vi "New.vi"(7 "id (0)":i32, 8 "error in (no error)":errorcluster, 9 "priority (100)":i32=100, 10 "processor (-2)":i32=-2, 11 "Thread type":refnum<class "Thread.lvclass">) -> (0 "error out":errorcluster, 3 "Thread":refnum<class "Thread.lvclass">)   [LabVIEW 2017, in "DSF Core.lvlib" / "Thread.lvclass"]
uses:
  Thread.lvclass
  Thread.lvclass/Thread.ctl
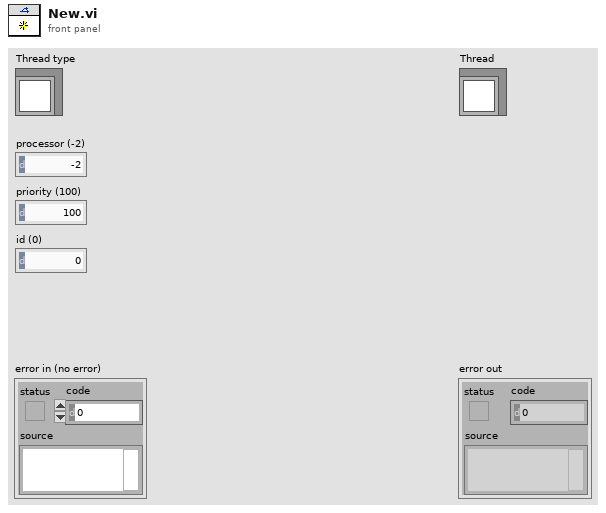
[diagram p1: front panel]
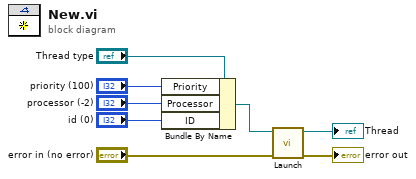
[diagram p0: block diagram]
diagram:
  n1 = Bundle By Name(cluster="Thread type", "Priority"="priority (100)", "Processor"="processor (-2)", "ID"="id (0)") -> (w1:refnum<class "Thread.lvclass">)
  n2 = call "Launch.vi"("error in (no error)"="error in (no error)", "Thread in"=w1) -> ("error out"=→"error out":errorcluster, "Thread out"=→"Thread":refnum<class "Thread.lvclass">)  [unwired: 8 in]
